vi "Initialize Constants.vi"(0 "option name/value pairs":cluster{"option":string, "value":string}[](array[cluster]), 11 "error in":errorcluster) -> (15 "error out":errorcluster)   [LabVIEW 2019]
uses:
  TypeDefs/Constants.ctl
  Global Constants.vi
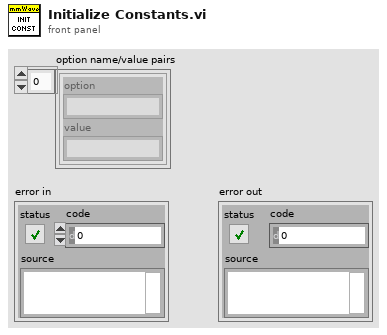
[diagram p1: front panel]
types:
  T1 = typedef "Constants.ctl" = cluster{"data clock rate (Hz)":dbl, "sample rate (Hz)":dbl, "sample rate selector string":string, "default tx bitfile path":path, "default rx bitfile path":path, "default proc bitfile path":path}
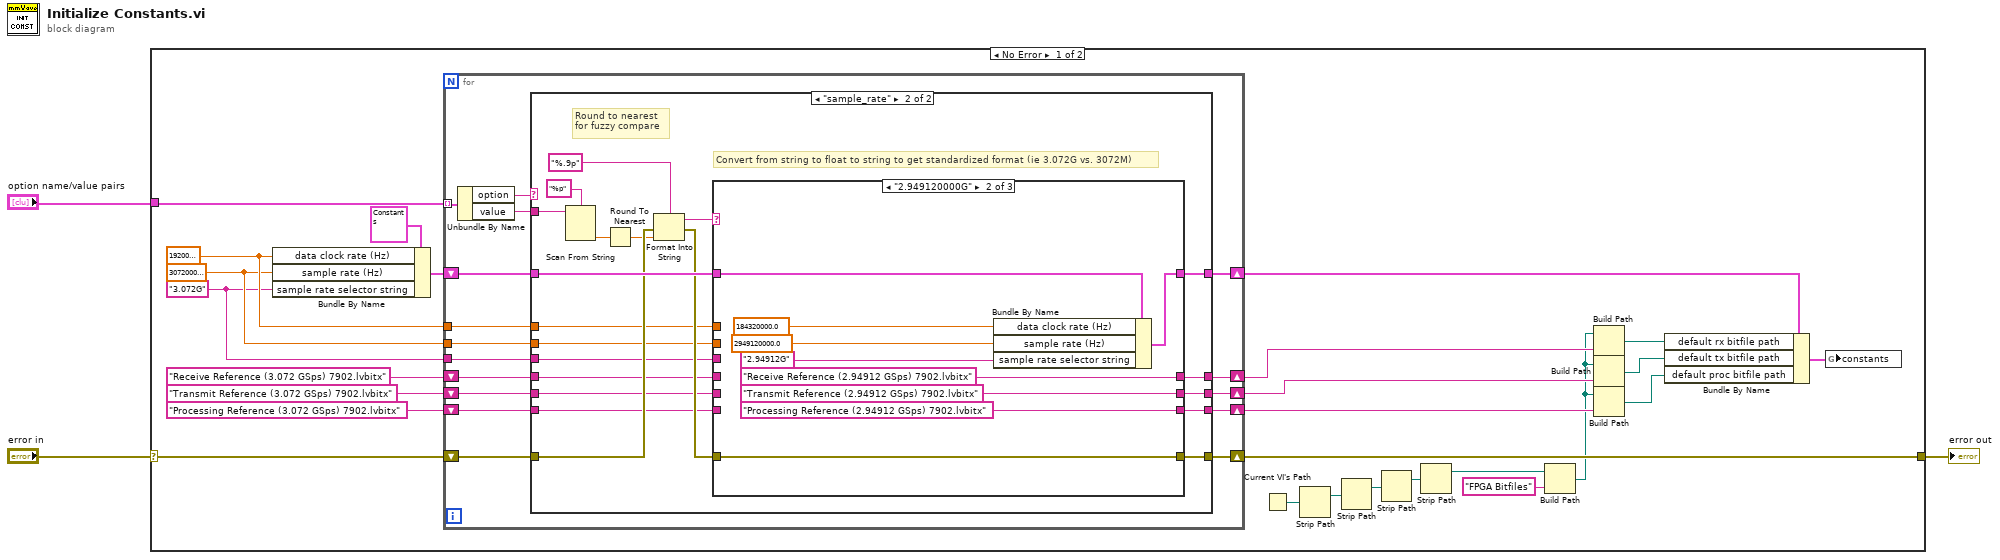
[diagram p0: block diagram]
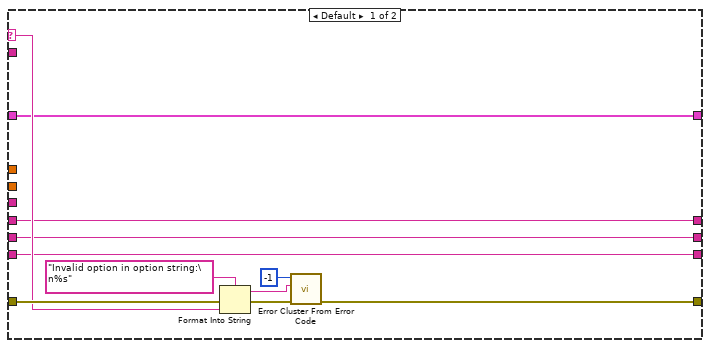
[diagram p2: hidden frame]
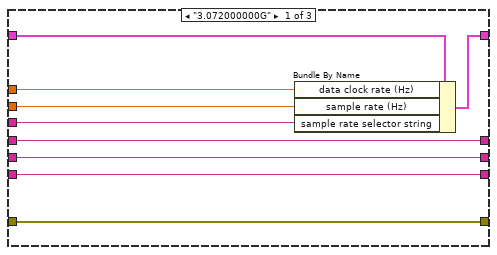
[diagram p3: hidden frame]
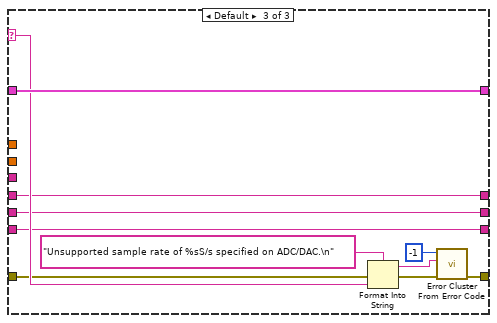
[diagram p4: hidden frame]
diagram:
  n1 = case shown="No Error" "error in" {
    selector: "error in" -> [w26 w106]
    tunnel: "option name/value pairs" -> [w27 _]
    tunnel: [w29 w106] -> w3
    frame No Error {
      w4 = "3.072G" ("sample rate selector string")
      w23 = 3072000000.0 ("sample rate (Hz)")
      w24 = 192000000.0 ("data clock rate (Hz)")
      n2 = Bundle By Name(cluster=T1 {"data clock rate (Hz)"=0.0, "sample rate (Hz)"=0.0, "sample rate selector string"="", "default tx bitfile path"=path "", "default rx bitfile path"=path "", "default proc bitfile path"=path ""} ("constants"), "data clock rate (Hz)"=w24, "sample rate (Hz)"=w23, "sample rate selector string"=w4) -> (w28:T1)
      n3 = for {
        shift-right: [w44] -> w29
        shift-left: w26 -> [w45]
        shift-right: [w42] -> w14
        shift-left: w28 -> [w43]
        tunnel: w24 -> [w41]
        tunnel: w23 -> [w40]
        tunnel: w27 -> [w39] mode=indexing
        shift-right: [w33] -> w10
        shift-left: "Transmit Reference (3.072 GSps) 7902.lvbitx" -> [w35]
        shift-right: [w34] -> w12
        shift-left: "Receive Reference (3.072 GSps) 7902.lvbitx" -> [w36]
        shift-right: [w31] -> w7
        shift-left: "Processing Reference (3.072 GSps) 7902.lvbitx" -> [w32]
        tunnel: w4 -> [w30]
        n4 = Unbundle By Name(w39) -> ("option"=w38:string, "value"=w37:string)
        n5 = case shown="\"sample_rate\"" w38 {
          selector: w38 -> [w50 _]
          tunnel: w37 -> [_ w76]
          tunnel: w45 -> [w52 w69]
          tunnel: [w54 w72] -> w44
          tunnel: w43 -> [w49 w73]
          tunnel: [w49 w71] -> w42
          tunnel: w41 -> [_ w67]
          tunnel: w40 -> [_ w66]
          tunnel: w36 -> [w48 w63]
          tunnel: w35 -> [w47 w62]
          tunnel: [w48 w61] -> w34
          tunnel: [w47 w60] -> w33
          tunnel: w32 -> [w46 w59]
          tunnel: [w46 w58] -> w31
          tunnel: w30 -> [_ w57]
          frame Default {
            n6 = Format Into String(format string="Invalid option in option string:\n%s" ("error message (\"\")"), error in=w52, w50) -> (resulting string=w56:string, error out=w51:errorcluster)  [unwired: 1 in]
            n7 = call <vilib>:"Error Cluster From Error Code.vi"("error in (no error)"=w51, "error message (\"\")"=w56, "error code (0)"=-1) -> ("error out"=w54:errorcluster)  [unwired: 6 in]
          }
          frame "sample_rate" {
            # "Round to nearest\nfor fuzzy compare"
            # "Convert from string to float to string to get standardized format (ie 3.072G vs. 3072M)"
            n8 = Scan From String(format string="%p", input string=w76) -> (output 1=w65:dbl)  [unwired: 3 in, 3 out]
            n9 = Round To Nearest(number=w65) -> (nearest integer value=w64:dbl)
            n10 = Format Into String(format string="%.9p", error in=w69, w64) -> (resulting string=w74:string, error out=w68:errorcluster)  [unwired: 1 in]
            n11 = case shown="\"2.949120000G\"" w74 {
              selector: w74 -> [_ _ w101]
              tunnel: w73 -> [w84 w93 w105]
              tunnel: w68 -> [w85 w94 w100]
              tunnel: [w85 w94 w99] -> w72
              tunnel: [w83 w92 w105] -> w71
              tunnel: w67 -> [w82 _ _]
              tunnel: w66 -> [w81 _ _]
              tunnel: w63 -> [w80 _ w97]
              tunnel: w62 -> [w79 _ w96]
              tunnel: [w80 "Receive Reference (2.94912 GSps) 7902.lvbitx" w97] -> w61
              tunnel: [w79 "Transmit Reference (2.94912 GSps) 7902.lvbitx" w96] -> w60
              tunnel: w59 -> [w78 _ w95]
              tunnel: [w78 "Processing Reference (2.94912 GSps) 7902.lvbitx" w95] -> w58
              tunnel: w57 -> [w77 _ _]
              frame "3.072000000G" {
                n12 = Bundle By Name(cluster=w84, "data clock rate (Hz)"=w82, "sample rate (Hz)"=w81, "sample rate selector string"=w77) -> (w83:T1)
              }
              frame "2.949120000G" {
                n13 = Bundle By Name(cluster=w93, "data clock rate (Hz)"=184320000.0, "sample rate (Hz)"=2949120000.0, "sample rate selector string"="2.94912G") -> (w92:T1)
              }
              frame Default {
                n14 = Format Into String(format string="Unsupported sample rate of %sS/s specified on ADC/DAC.\n" ("error message (\"\")"), error in=w100, w101) -> (resulting string=w104:string, error out=w102:errorcluster)  [unwired: 1 in]
                n15 = call <vilib>:"Error Cluster From Error Code.vi"("error in (no error)"=w102, "error message (\"\")"=w104, "error code (0)"=-1) -> ("error out"=w99:errorcluster)  [unwired: 6 in]
              }
            }
          }
        }
      }
      n16 = Current VI's Path() -> (path=w22:path)
      n17 = Strip Path(path=w22) -> (stripped path=w21:path)  [unwired: 1 out]
      n18 = Strip Path(path=w21) -> (stripped path=w20:path)  [unwired: 1 out]
      n19 = Strip Path(path=w20) -> (stripped path=w19:path)  [unwired: 1 out]
      n20 = Strip Path(path=w19) -> (stripped path=w17:path)  [unwired: 1 out]
      n21 = Build Path(base path=w17, name or relative path="FPGA Bitfiles") -> (appended path=w6:path)
      n22 = Build Path(base path=w6, name or relative path=w12) -> (appended path=w11:path)
      n23 = Build Path(base path=w6, name or relative path=w10) -> (appended path=w9:path)
      n24 = Build Path(base path=w6, name or relative path=w7) -> (appended path=w5:path)
      n25 = Bundle By Name(cluster=w14, "default rx bitfile path"=w11, "default tx bitfile path"=w9, "default proc bitfile path"=w5) -> (w13:T1)
      n26 = global write "Global Constants.vi" "constants"(w13) -> ()
    }
    frame Error {
    }
  }
  "error out" <- w3
